vi "FPGA Main.vi"() -> ()   [LabVIEW 2013]
uses:
  <vilib>/eio/EIOMethodNode/EIOMethodNode.xnode
  <vilib>/rvi/eio/common/nirviEmuTemplateMethod_errors.vi
  <vilib>/eio/EIOPropertyNode/EIOPropertyNode.xnode
  <vilib>/rvi/eio/common/nirviEmuTemplatePropertyGet_errors.vi
  <vilib>/rvi/eio/common/nirviEmuTemplatePropertyGet_noerrors.vi
  <vilib>/rvi/eio/common/nirviEmuTemplatePropertySet_errors.vi
  <vilib>/rvi/eio/common/nirviEmuTemplatePropertySet_noerrors.vi
panel:
  in  "cRIO-PB Properties":bool
  in  "HostRequest":bool
  out "GetData":u8
  out "DataLen":u8
  in  "Mode":T1(ring)
  in  "ByteIndex":u8
  in  "SetData":u8
  out "Status":u8 format="%.0x"
  in  "Slave/Service":i8
  out "SerialNumber":u32
  out "ModuleID":u16 format="%.0x"
  out "VendorID":u16 format="%.0x"
  in  "Stop":bool
  out "Error":errorcluster
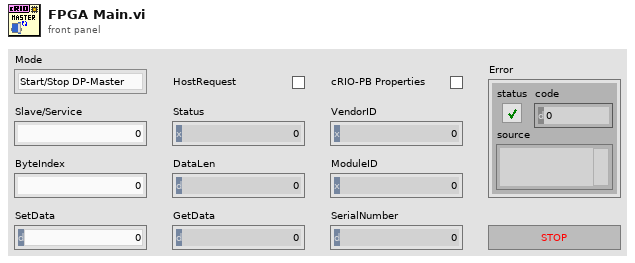
[diagram p1: front panel]
types:
  T1 = enum16{"Start/Stop DP-Master", "Get Input Data", "Set Output Data", "Get Output Data", "Get Diagnostic Data", "Read/Write Data", "Read Diagnostic Data", "Get DPV1 Data", "Set DPV1 Data", "Read/Write DPV1 Data"}
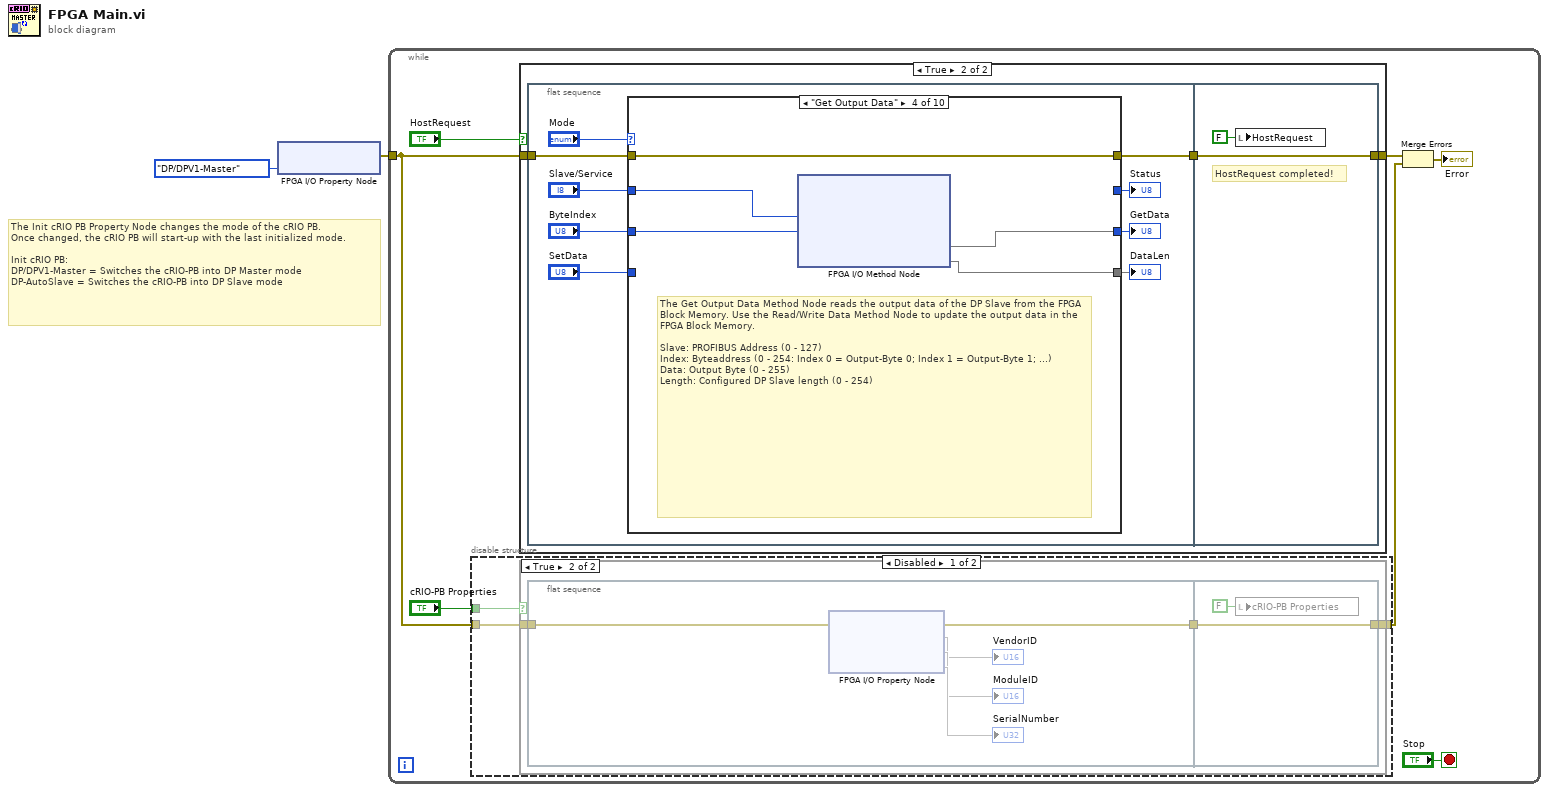
[diagram p0: block diagram]
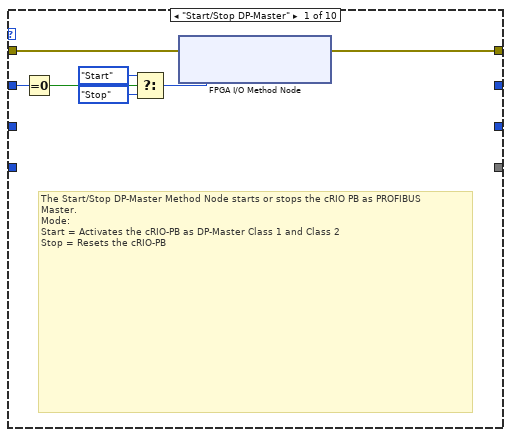
[diagram p5: hidden frame]
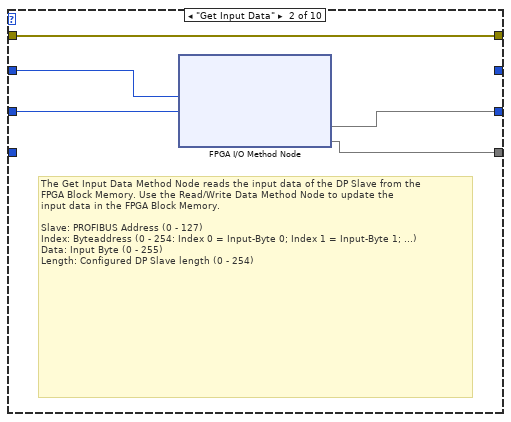
[diagram p6: hidden frame]
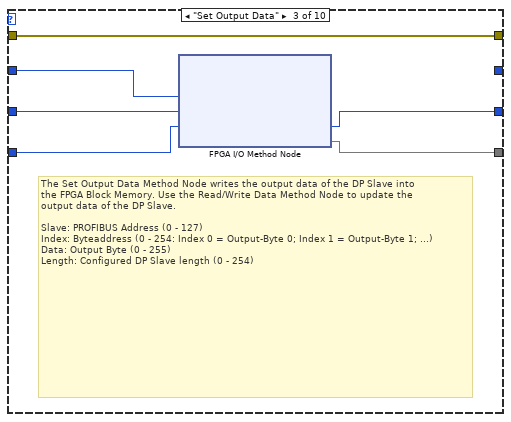
[diagram p7: hidden frame]
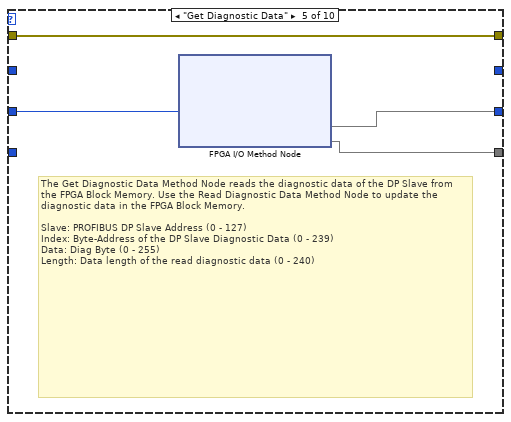
[diagram p8: hidden frame]
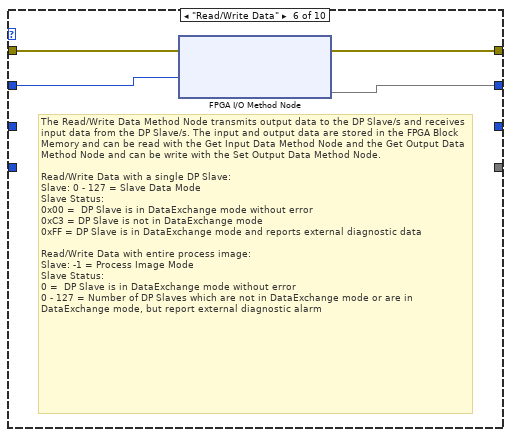
[diagram p9: hidden frame]
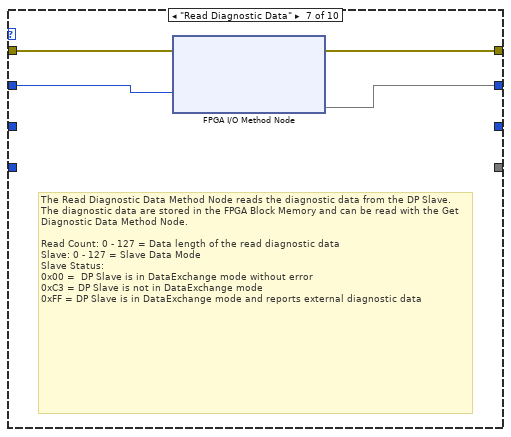
[diagram p10: hidden frame]
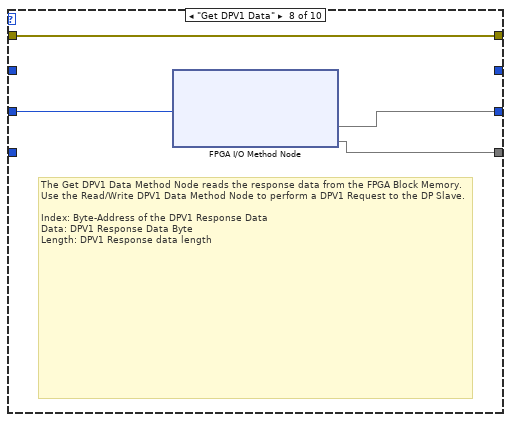
[diagram p11: hidden frame]
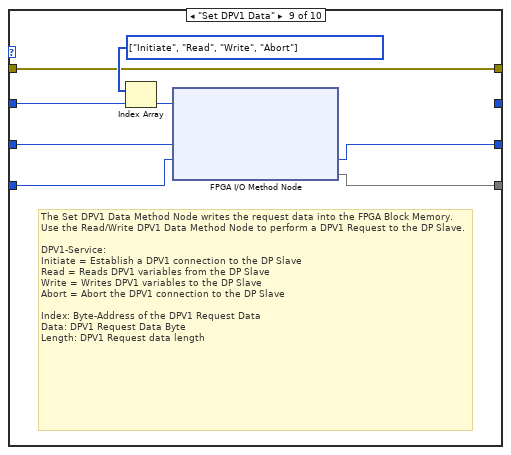
[diagram p12: hidden frame]
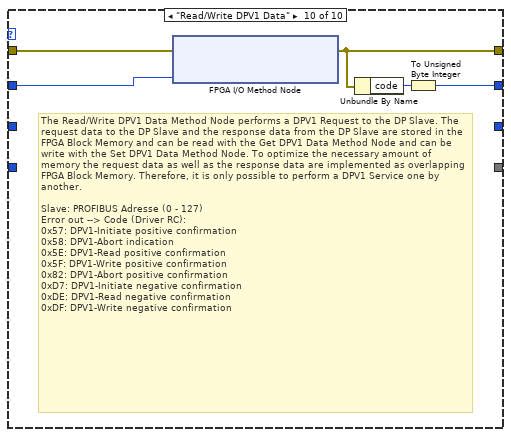
[diagram p13: hidden frame]
diagram:
  # "The Init cRIO PB Property Node changes the mode of the cRIO PB. \nOnce changed, the cRIO PB will start-up with the last initialized mode.\n\nInit cRIO PB: \nDP/DPV1-Master\t= Switches the cRIO-PB into DP Master mode\nDP-AutoSlave =\tSwitches the cRIO-PB into DP Slave mode"
  n1 = xnode "FPGA I/O Property Node"("Init cRIO PB"=enum8{"DP/DPV1-Master", "DP-AutoSlave"}."DP/DPV1-Master" ("Start-up cRIO PB")) -> ("error out"=w1:errorcluster)  [unwired: 2 in, 1 out]
  n2 = while {
    tunnel: w1 -> [w3]
    stop <- "Stop" stop-if-true
    n3 = disable-structure shown="Disabled" {
      disable-tunnel: "cRIO-PB Properties" -> [w12 _]
      disable-tunnel: [w11 _] -> w4
      disable-tunnel: w3 -> [w10 _]
      frame Disabled {
        n4 = case shown="True" w12 {
          tunnel: [w13 w15] -> w11
          tunnel: w10 -> [w13 w14]
          frame False {
          }
          frame True {
            n5 = flat-sequence {
              tunnel: [w18] -> w16
              tunnel: w14 -> [w17]
              tunnel: w16 -> [w22]
              tunnel: [w22] -> w15
              frame #0 {
                n6 = xnode "FPGA I/O Property Node"("error in"=w17) -> ("error out"=w18:errorcluster, "Vendor ID"=→"VendorID", "Module ID"=→"ModuleID", "Serial Number"=→"SerialNumber")  [unwired: 1 in, 1 out]
              }
              frame #1 {
                n7 = local write "cRIO-PB Properties"(FALSE ("SetData")) -> ()
              }
            }
          }
        }
      }
      frame Enabled {
      }
    }
    n8 = case shown="True" "HostRequest" {
      tunnel: w3 -> [w24 w27]
      tunnel: [w24 w26] -> w8
      frame False {
        # "Wait for new HostRequest!"
      }
      frame True {
        n9 = flat-sequence {
          tunnel: w27 -> [w29]
          tunnel: [w28] -> w25
          tunnel: [w88] -> w26
          tunnel: w25 -> [w88]
          frame #0 {
            n10 = case shown="\"Get Output Data\"" "Mode" {
              tunnel: "ByteIndex" -> [_ w48 w52 w57 w62 _ _ w72 w78 _]
              tunnel: [_ w45 w50 w56 w61 _ _ w73 w75 _] -> w33
              tunnel: [_ w46 w51 w55 w60 _ _ w74 w79 _] -> w32
              tunnel: "Slave/Service" -> [w37 w47 w53 w58 _ w66 w68 _ w76 w85]
              tunnel: "SetData" -> [_ _ w50 _ _ _ _ _ w75 _]
              tunnel: [_ _ _ _ _ w65 w67 _ _ w82] -> w30
              tunnel: w29 -> [w42 w44 w49 w54 w59 w64 w70 w71 w80 w86]
              tunnel: [w41 w44 w49 w54 w59 w63 w69 w71 w80 w84] -> w28
              frame "Start/Stop DP-Master" {
                # "The Start/Stop DP-Master Method Node starts or stops the cRIO PB as PROFIBUS \nMaster.\nMode: \nStart = Activates the cRIO-PB as DP-Master Class 1 and Class 2\nStop = Resets the cRIO-PB"
                n11 = Equal To 0?(x=w37) -> (x = 0?=w43:bool)
                n12 = Select(t=enum16{"Start", "Stop"}."Start" ("Mode"), s=w43, f=enum16{"Start", "Stop"}."Stop" ("Mode")) -> (s? t:f=w38:enum16{"Start", "Stop"})
                n13 = xnode "FPGA I/O Method Node"("error in"=w42, "Mode"=w38) -> ("error out"=w41:errorcluster)  [unwired: 1 in, 1 out]
              }
              frame "Get Input Data" {
                # "The Get Input Data Method Node reads the input data of the DP Slave from the \nFPGA Block Memory. Use the Read/Write Data Method Node to update the \ninput data in the FPGA Block Memory.\n\nSlave: PROFIBUS Address (0 - 127)\nIndex: Byteaddress (0 - 254: Index 0 = Input-Byte 0; Index 1 = Input-Byte 1; ...)\nData: Input Byte (0 - 255)\nLength: Configured DP Slave length (0 - 254)"
                n14 = xnode "FPGA I/O Method Node"("Slave"=w47, "Index"=w48) -> ("Data"=w45, "Length"=w46)  [unwired: 1 in, 1 out]
              }
              frame "Set Output Data" {
                # "The Set Output Data Method Node writes the output data of the DP Slave into \nthe FPGA Block Memory. Use the Read/Write Data Method Node to update the \noutput data of the DP Slave.\n\nSlave: PROFIBUS Address (0 - 127)\nIndex: Byteaddress (0 - 254: Index 0 = Output-Byte 0; Index 1 = Output-Byte 1; ...)\nData: Output Byte (0 - 255)\nLength: Configured DP Slave length (0 - 254)"
                n15 = xnode "FPGA I/O Method Node"("Slave"=w53, "Index"=w52, "Data"=w50) -> ("Length"=w51)  [unwired: 1 in, 1 out]
              }
              frame "Get Output Data" {
                # "The Get Output Data Method Node reads the output data of the DP Slave from the FPGA Block Memory. Use the Read/Write Data Method Node to update the output data in the FPGA Block Memory.\n\nSlave: PROFIBUS Address (0 - 127)\nIndex: Byteaddress (0 - 254: Index 0 = Output-Byte 0; Index 1 = Output-Byte 1; ...)\nData: Output Byte (0 - 255)\nLength: Configured DP Slave length (0 - 254)"
                n16 = xnode "FPGA I/O Method Node"("Slave"=w58, "Index"=w57) -> ("Data"=w56, "Length"=w55)  [unwired: 1 in, 1 out]
              }
              frame "Get Diagnostic Data" {
                # "The Get Diagnostic Data Method Node reads the diagnostic data of the DP Slave from the FPGA Block Memory. Use the Read Diagnostic Data Method Node to update the diagnostic data in the FPGA Block Memory.\n\nSlave:\tPROFIBUS DP Slave Address\t(0 - 127)\nIndex:\tByte-Address of the DP Slave Diagnostic Data (0 - 239)\nData:\tDiag Byte\t(0 - 255)\nLength:\tData length of the read diagnostic data\t(0 - 240)"
                n17 = xnode "FPGA I/O Method Node"("Index"=w62) -> ("Data"=w61, "Length"=w60)  [unwired: 1 in, 2 out]
              }
              frame "Read/Write Data" {
                # "The Read/Write Data Method Node transmits output data to the DP Slave/s and receives input data from the DP Slave/s. The input and output data are stored in the FPGA Block Memory and can be read with the Get Input Data Method Node and the Get Output Data Method Node and can be write with the Set Output Data Method Node.\n\nRead/Write Data with a single DP Slave:\nSlave:\t0 - 127 = Slave Data Mode \nSlave Status:\t\n0x00 = \tDP Slave is in DataExchange mode without error\n0xC3 =\tDP Slave is not in DataExchange mode \n0xFF =\tDP Slave is in DataExchange mode and reports external diagnostic data\n \nRead/Write Data with entire process image:\nSlave: -1 = Process Image Mode\nSlave Status:\t\n0 = \tDP Slave is in DataExchange mode without error\n0 - 127 = Number of DP Slaves which are not in DataExchange mode or are in DataExchange mode, but report external diagnostic alarm"
                n18 = xnode "FPGA I/O Method Node"("error in"=w64, "Slave"=w66) -> ("error out"=w63:errorcluster, "Slave Status"=w65)  [unwired: 1 in, 1 out]
              }
              frame "Read Diagnostic Data" {
                # "The Read Diagnostic Data Method Node reads the diagnostic data from the DP Slave. The diagnostic data are stored in the FPGA Block Memory and can be read with the Get Diagnostic Data Method Node.\n\nRead Count:\t0 - 127 = Data length of the read diagnostic data \nSlave:\t0 - 127 = Slave Data Mode \nSlave Status:\t\n0x00 = \tDP Slave is in DataExchange mode without error\n0xC3 =\tDP Slave is not in DataExchange mode \n0xFF =\tDP Slave is in DataExchange mode and reports external diagnostic data"
                n19 = xnode "FPGA I/O Method Node"("error in"=w70, "Slave"=w68) -> ("error out"=w69:errorcluster, "Slave Status"=w67)  [unwired: 1 in, 2 out]
              }
              frame "Get DPV1 Data" {
                # "The Get DPV1 Data Method Node reads the response data from the FPGA Block Memory. Use the Read/Write DPV1 Data Method Node to perform a DPV1 Request to the DP Slave.\n\nIndex:\tByte-Address of the DPV1 Response Data\nData:\tDPV1 Response Data Byte\nLength:\tDPV1 Response data length"
                n20 = xnode "FPGA I/O Method Node"("Index"=w72) -> ("Data"=w73, "Length"=w74)  [unwired: 1 in, 1 out]
              }
              frame "Set DPV1 Data" {
                w81 = enum8{"Initiate", "Read", "Write", "Abort"}[] [enum."Initiate", enum."Read", enum."Write", enum."Abort"] items=["Initiate", "Read", "Write", "Abort"]
                # "The Set DPV1 Data Method Node writes the request data into the FPGA Block Memory. Use the Read/Write DPV1 Data Method Node to perform a DPV1 Request to the DP Slave.\n\nDPV1-Service:\t\nInitiate =\tEstablish a DPV1 connection to the DP Slave\nRead =\tReads DPV1 variables from the DP Slave\nWrite =\tWrites DPV1 variables to the DP Slave\nAbort =\tAbort the DPV1 connection to the DP Slave\n\nIndex:\tByte-Address of the DPV1 Request Data\nData:\tDPV1 Request Data Byte\nLength:\tDPV1 Request data length"
                n21 = Index Array(array=w81, index=w76) -> (element=w77:enum8{"Initiate", "Read", "Write", "Abort"})
                n22 = xnode "FPGA I/O Method Node"("DPV1-Service"=w77, "Index"=w78, "Data"=w75) -> ("Length"=w79)  [unwired: 1 in, 1 out]
              }
              frame "Read/Write DPV1 Data" {
                # "The Read/Write DPV1 Data Method Node performs a DPV1 Request to the DP Slave. The request data to the DP Slave and the response data from the DP Slave are stored in the FPGA Block Memory and can be read with the Get DPV1 Data Method Node and can be write with the Set DPV1 Data Method Node. To optimize the necessary amount of memory the request data as well as the response data are implemented as overlapping FPGA Block Memory. Therefore, it is only possible to perform a DPV1 Service one by another.\n\nSlave: PROFIBUS Adresse (0 - 127)\nError out --> Code (Driver RC): \n0x57: DPV1-Initiate positive confirmation\n0x58: DPV1-Abort indication\n0x5E: DPV1-Read positive confirmation\n0x5F: DPV1-Write positive confirmation\n0x82: DPV1-Abort positive confirmation\n0xD7: DPV1-Initiate negative confirmation\n0xDE: DPV1-Read negative confirmation\n0xDF: DPV1-Write negative confirmation"
                n23 = xnode "FPGA I/O Method Node"("error in"=w86, "Slave"=w85) -> ("error out"=w84:errorcluster)  [unwired: 1 in, 1 out]
                n24 = Unbundle By Name(w84) -> ("code"=w83:i32)
                n25 = To Unsigned Byte Integer(number=w83) -> (unsigned 8bit integer=w82:u8)
              }
            }
            "DataLen" <- w32
            "GetData" <- w33
            "Status" <- w30
          }
          frame #1 {
            # "HostRequest completed!"
            n26 = local write "HostRequest"(FALSE ("SetData")) -> ()
          }
        }
      }
    }
    n27 = Merge Errors(w8, w4) -> (→"Error":errorcluster)
  }
